vi "XIPIN_AXI_GPIO_2_0.vi"   [LabVIEW 2017]
doc: "Advanced eXtensible Interface General Purpose Input/Output (AXI GPIO) core provides a general purpose input/output interface to the AXI interface.\n------------------------------------\n<b>Need License</b> : No\n<b>Interface</b> : AXI4"
uses:
  <vilib>/rvi/XilinxIP/XIPIN_XNode/niFpgaXIPIN.xnode
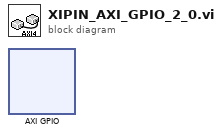
[diagram p0: block diagram]
diagram:
  n1 = xnode ("AXI GPIO")() -> ()
